vi "Read database.vi"(5 "String":string) -> (0 "error out":errorcluster, 2 "DB Data":T1)   [LabVIEW 2015]
uses:
  <vilib>/addons/database/Connection.llb/DB Tools Open Connec (String).vi
  Galobal variable_TI.vi
  <vilib>/addons/database/_DB Variant To Data/Database Variant To Data.xnode
  <vilib>/addons/database/NI_Database_API.lvlib
panel:
  out "appended array 4":string[](array[string])
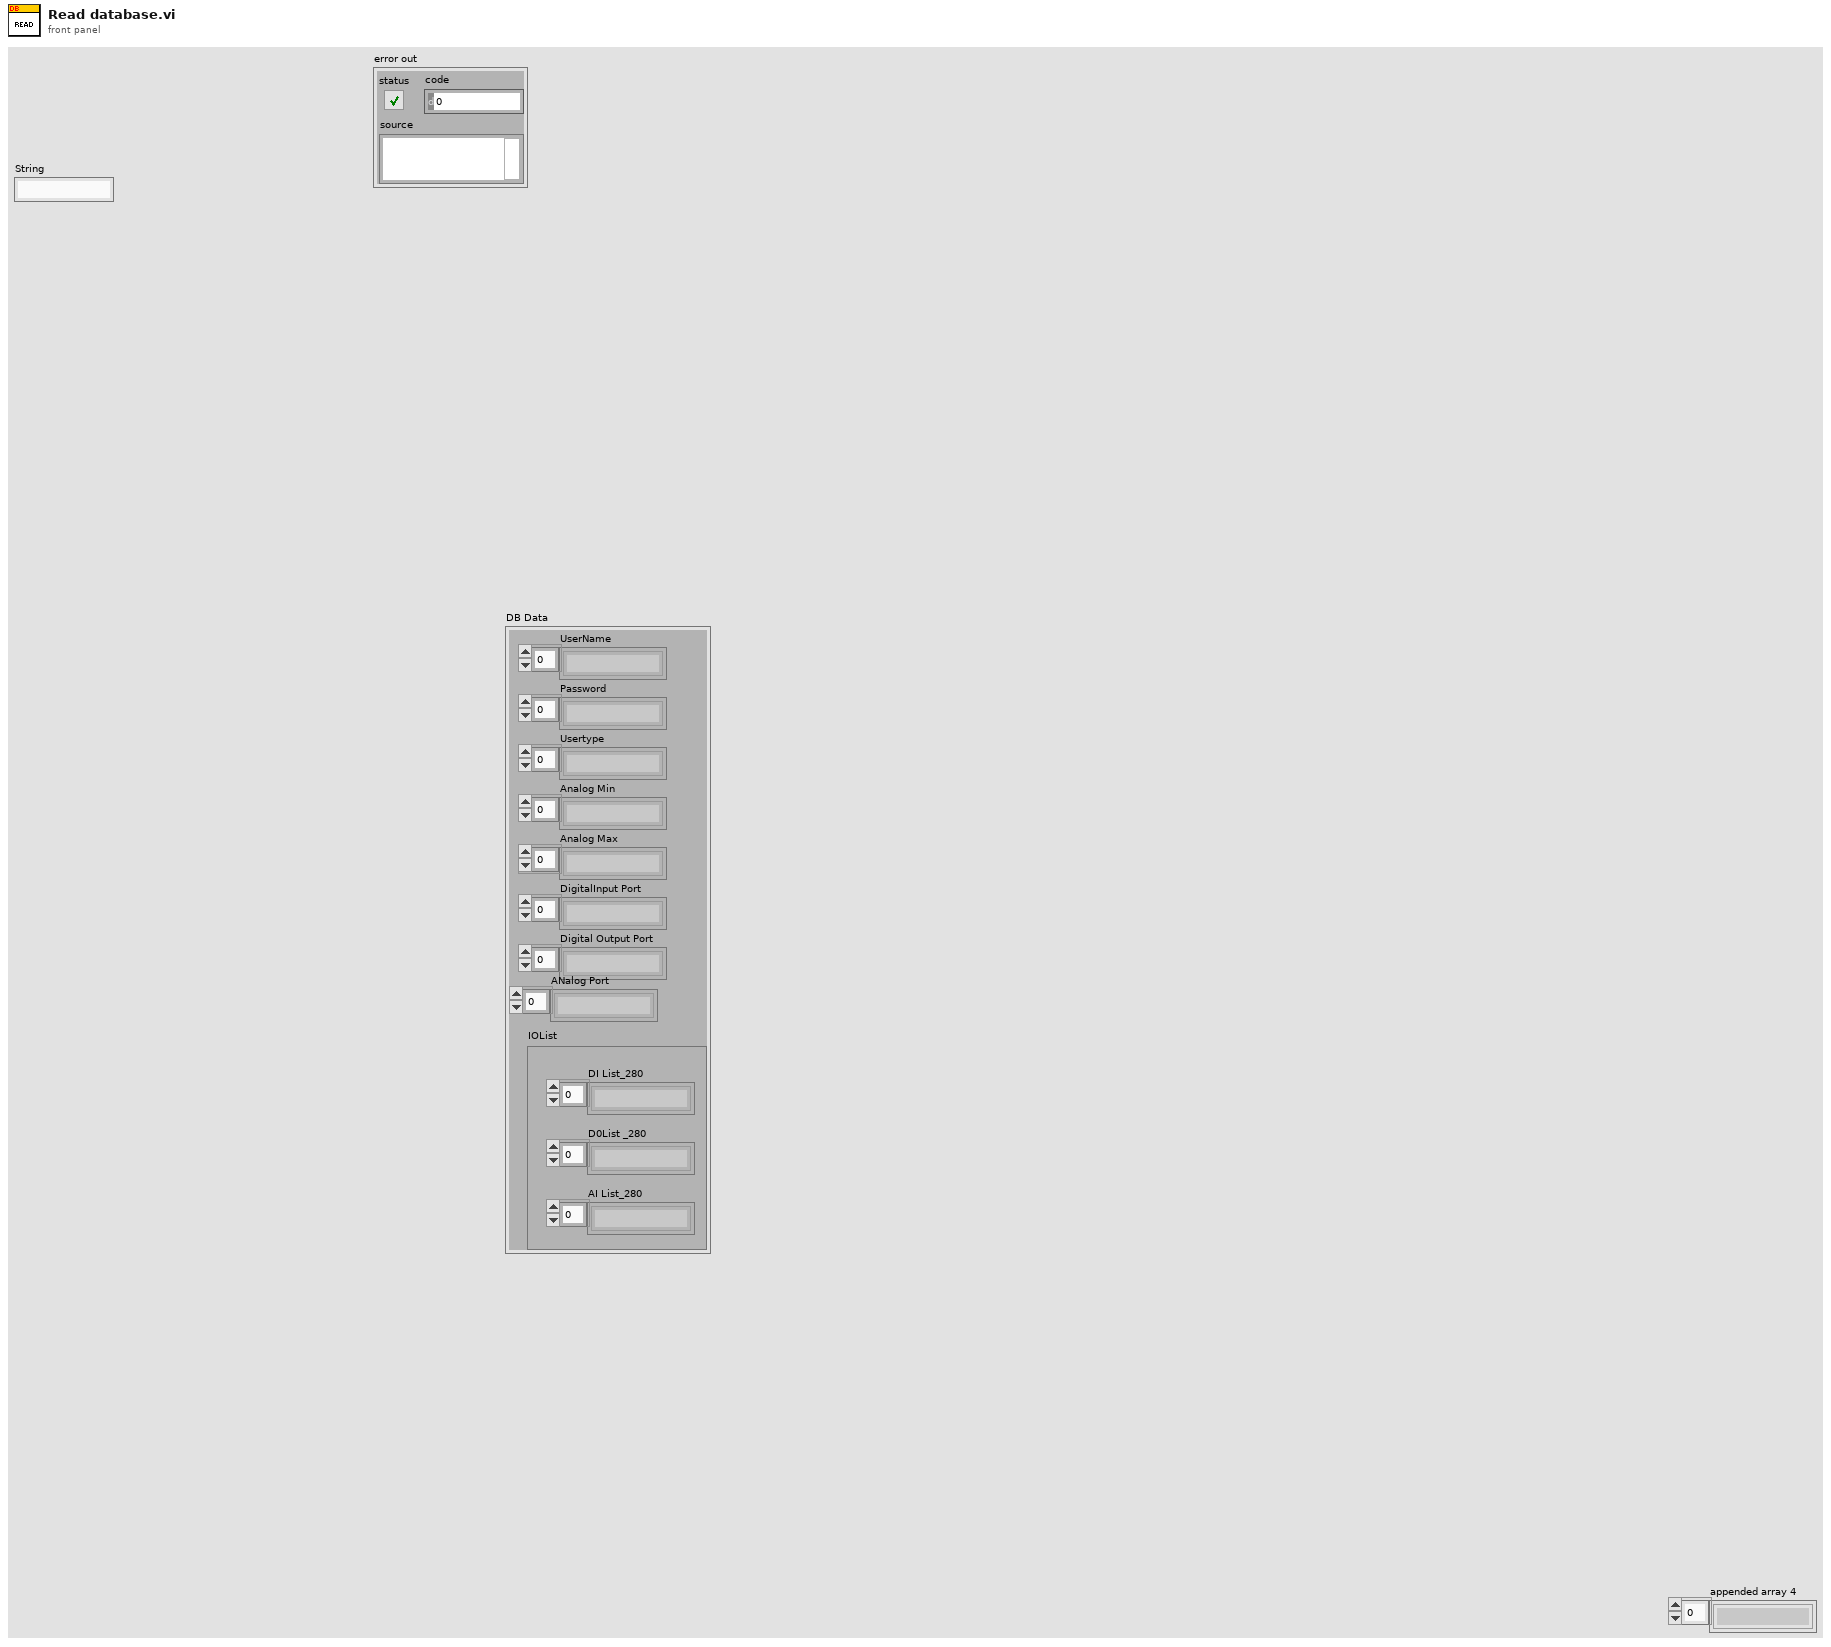
[diagram p1: front panel]
types:
  T1 = cluster{"UserName":string[], "Password":string[], "Usertype":string[], "Analog Min":string[], "Analog Max":string[], "DigitalInput Port":string[], "Digital Output Port":string[], "ANalog Port":string[], "IOList":cluster{"DI List_280":string[], "D0List _280":string[], "AI List_280":string[]}}
  T2 = cluster{"To-A":timestamp, "From-A":timestamp, "From-B":timestamp, "To-B":timestamp, "From-C":timestamp, "To-C":timestamp, "Shift":string}[]
  T3 = typedef "NI_Database_API.lvlib/Conn ObjectReference.ctl" = refnum<k1>
  T4 = cluster{"DI List_280":string[], "D0List _280":string[], "AI List_280":string[]}
  T5 = cluster{"To-A":timestamp, "From-A":timestamp, "From-B":timestamp, "To-B":timestamp, "From-C":timestamp, "To-C":timestamp, "Shift":string}
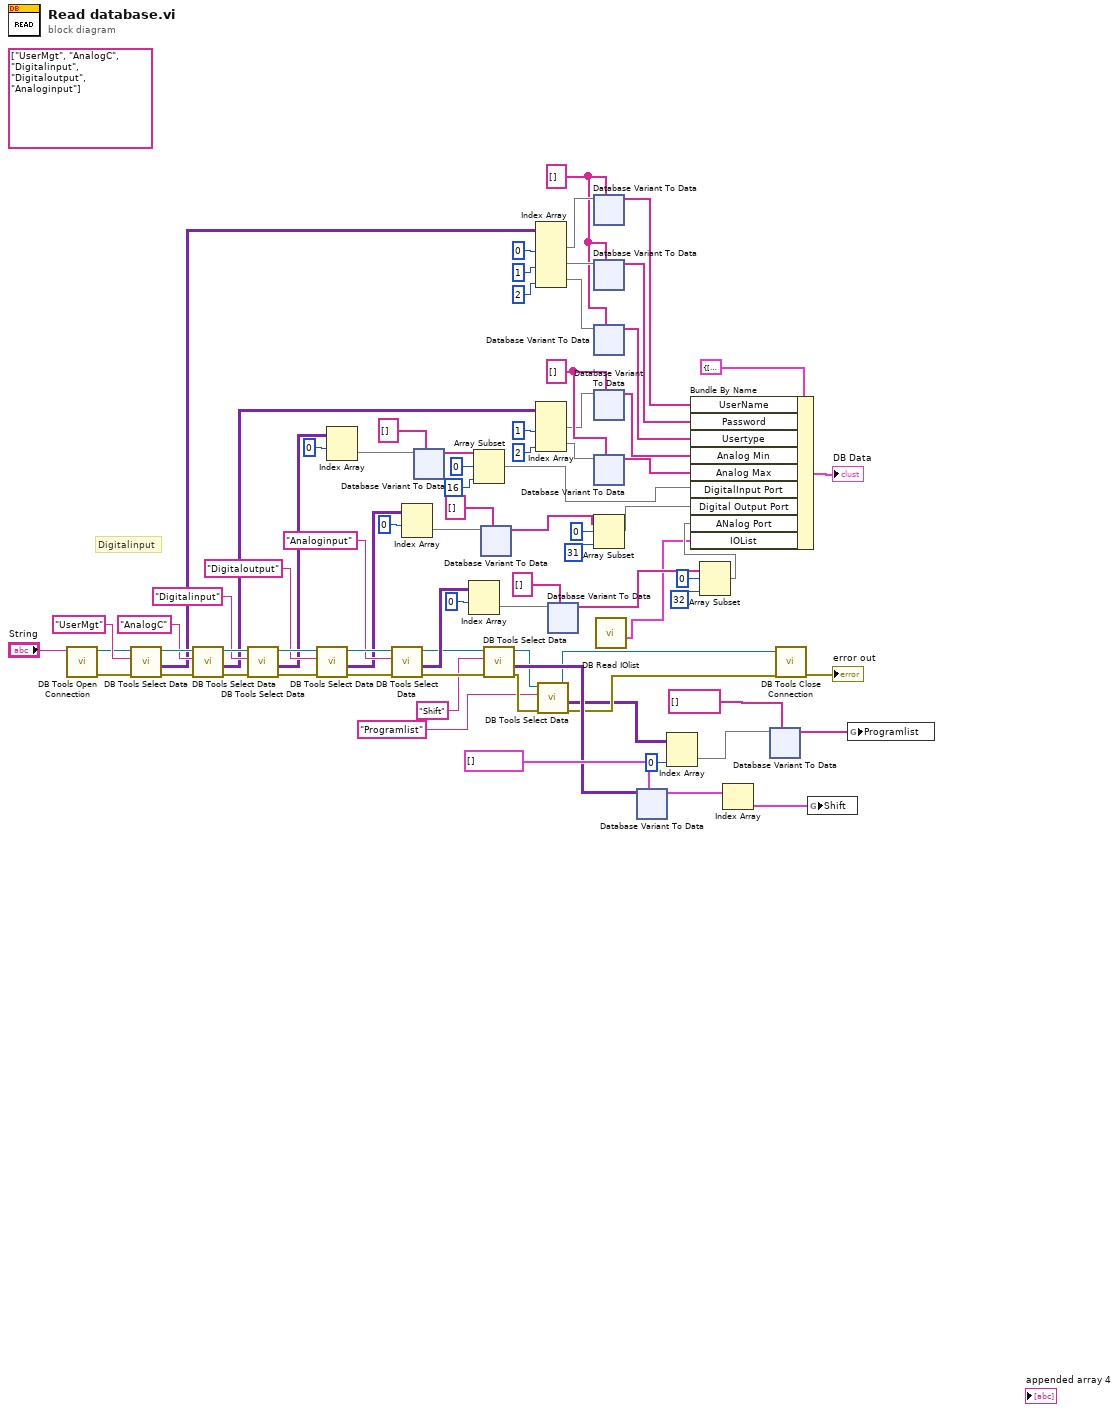
[diagram p0: block diagram]
diagram:
  w71 = string[] []
  (unwired) string[] ["UserMgt", "AnalogC", "Digitalinput", "Digitaloutput", "Analoginput"]
  w60 = string[] []
  # "Digitalinput"
  n1 = call-poly <vilib>:"DB Tools Open Connection.vi"("connection information"="String") -> ("error out"=w38:errorcluster, "connection reference"=w39:T3)  [unwired: 7 in]
  n2 = call <vilib>:"DB Tools Select Data.vi"("error in (no error)"=w38, "table"="UserMgt", "connection reference"=w39) -> ("error out"=w52:errorcluster, "data"=w37:variant[][], "connection reference out"=w50:T3)  [unwired: 3 in]
  n3 = call <vilib>:"DB Tools Select Data.vi"("error in (no error)"=w52, "table"="AnalogC", "connection reference"=w50) -> ("error out"=w51:errorcluster, "data"=w36:variant[][], "connection reference out"=w49:T3)  [unwired: 3 in]
  n4 = call <vilib>:"DB Tools Select Data.vi"("error in (no error)"=w51, "table"="Digitalinput", "connection reference"=w49) -> ("error out"=w45:errorcluster, "data"=w35:variant[][], "connection reference out"=w44:T3)  [unwired: 3 in]
  n5 = call <vilib>:"DB Tools Select Data.vi"("error in (no error)"=w45, "table"="Digitaloutput", "connection reference"=w44) -> ("error out"=w41:errorcluster, "data"=w34:variant[][], "connection reference out"=w42:T3)  [unwired: 3 in]
  n6 = Index Array(array=w35, index (row)=0 ("disabled index (col)")) -> (element=w73:variant[])  [unwired: 1 in]
  n7 = call <vilib>:"DB Tools Select Data.vi"("error in (no error)"=w41, "table"="Analoginput", "connection reference"=w42) -> ("error out"=w28:errorcluster, "data"=w33:variant[][], "connection reference out"=w27:T3)  [unwired: 3 in]
  n8 = Index Array(array=w34, index (row)=0 ("disabled index (col)")) -> (element=w74:variant[])  [unwired: 1 in]
  n9 = xnode "Database Variant To Data"("database variant"=w73, "type"=string[] []) -> ("data"=w23:string[])  [unwired: 1 in, 1 out]
  n10 = Index Array(array=w33, index (row)=0 ("disabled index (col)")) -> (element=w77:variant[])  [unwired: 1 in]
  n11 = Array Subset(array=w23, index=0, length=16) -> (w20:string[])
  n12 = xnode "Database Variant To Data"("database variant"=w74, "type"=string[] []) -> ("data"=w18:string[])  [unwired: 1 in, 1 out]
  n13 = call <vilib>:"DB Tools Select Data.vi"("error in (no error)"=w28, "table"="Shift", "connection reference"=w27) -> ("error out"=w9:errorcluster, "data"=w25:variant[][], "connection reference out"=w10:T3)  [unwired: 3 in]
  n14 = Index Array(array=w37, index (col) #1=0 ("disabled index (col)"), index (col) #2=1 ("index (col)"), index (col) #3=2 ("index (col)")) -> (element #1=w64:variant[], element #2=w61:variant[], element #3=w59:variant[])  [unwired: 3 in]
  n15 = Index Array(array=w36, index (col) #1=1 ("disabled index (col)"), index (col) #2=2 ("index (col)")) -> (element #1=w69:variant[], element #2=w70:variant[])  [unwired: 2 in]
  n16 = call <vilib>:"DB Tools Select Data.vi"("error in (no error)"=w9, "table"="Programlist", "connection reference"=w10) -> ("error out"=w6:errorcluster, "data"=w5:variant[][], "connection reference out"=w7:T3)  [unwired: 3 in]
  n17 = xnode "Database Variant To Data"("database variant"=w77, "type"=string[] []) -> ("data"=w13:string[])  [unwired: 1 in, 1 out]
  n18 = xnode "Database Variant To Data"("database variant"=w64, "type"=w60) -> ("data"=w58:string[])  [unwired: 1 in, 1 out]
  n19 = xnode "Database Variant To Data"("database variant"=w61, "type"=w60) -> ("data"=w57:string[])  [unwired: 1 in, 1 out]
  n20 = xnode "Database Variant To Data"("database variant"=w59, "type"=w60) -> ("data"=w56:string[])  [unwired: 1 in, 1 out]
  n21 = xnode "Database Variant To Data"("database variant"=w69, "type"=w71) -> ("data"=w55:string[])  [unwired: 1 in, 1 out]
  n22 = xnode "Database Variant To Data"("database variant"=w70, "type"=w71) -> ("data"=w54:string[])  [unwired: 1 in, 1 out]
  n23 = Array Subset(array=w18, index=0, length=31) -> (w16:string[])
  n24 = call "DB Read IOlist.vi"() -> ("output cluster"=w11:T4)  [unwired: 11 in]
  n25 = xnode "Database Variant To Data"("database variant"=w25, "type"=T2 []) -> ("data"=w29:T2)  [unwired: 1 in, 1 out]
  n26 = Index Array(array=w5, index (col)=0 ("disabled index (col)")) -> (element=w4:variant[])  [unwired: 1 in]
  n27 = Array Subset(array=w13, index=0, length=32) -> (w12:string[])
  n28 = Bundle By Name(cluster=T1 {"UserName"=[], "Password"=[], "Usertype"=[], "Analog Min"=[], "Analog Max"=[], "DigitalInput Port"=[], "Digital Output Port"=[], "ANalog Port"=[], "IOList"={"DI List_280"=[" Start PB (P0.0) ", "Emergency Stop (P0.1)", "Reset PB (P0.2)", "Home PB (P0.3)", "Main Pressure Signal (P0.4)", "Safety Signal-1 (P0.5)", "Safety Signal-2 (P0.6)", "Fixture Sliding Servo Home RS (P0.7)", "Fixture Sliding Servo Fault Signal (P0.8)", "LCD pressing Servo Home RS (P0.9)", "LCD pressing Servo fault Signal (P0.10)", "Spare", "Spare", "Spare", "Spare", "Model conformation PX-1 (AI2)", "Model conformation PX-2 (AI3)", "Diffuser height checking Sensor-1 (AI4)", "Diffuser height checking Sensor-2 (AI5)", "Panel Door Open Signal (AI6)", "Component CNF Sensor on Ionizer (AI7)", "Bi-adhesive tube Waste Collection bin CNF Sensor (AI8)", "Photo Prism presence Sensor (AI9)", "Lightbox presence CNF Sensor (AI10)", "Diffuser presence CNF Sensor (AI11)", "Photo prism height checking UP CYL Rs (AI12)", "Photo prism height checking DWN CYL  Rs (AI13)", "Camera slide Cyl Fwd Rs (AI14)", "Camera slide Cyl Rev Rs (AI15)", "LCD Display Rotating Unit Actuator Cyl CW PX (AI16)", "LCD Display Rotating Unit Actuator Cyl CCW PX (AI17)", "Fixture clamping Cyl Fwd Rs (AI18)", "Fixture clamping Cyl Rev Rs (AI19)", "Clip pulling unit Cyl Fwd Rs (AI20)", "Clip pulling unit Cyl Rev Rs (AI21)", "Clip clamp unit Cyl Fwd Rs (A22)", "Clip clamp unit Cyl Rev Rs (AI23)", "Barcode Scanner Ready Signal (AI24)", "Spare", "Spare", "Spare", "Spare", "Spare", "Spare", "Spare"], "D0List _280"=["Ionizer ON Sol (P0.16)", "Fixture Slide Servo Fault Reset (P0.17)", "LCD pressing servo Fault Reset (P0.18)", "Fixture Slide servo Brake ON Cmd (P0.19)", "Fixture Slide Servo Direction Command (P0.20)", "LCD pressing Servo Direction Command (P0.21)", "LCD pressing Servo Brake ON Cmd (P0.22)", "Photo prism height checking UP CYL Sol (P0.23)", "Photo prism height checking DWN CYL  Sol (P0.24)", "Camera slide Cyl Fwd Sol (P0.25)", "Camera slide Cyl Rev Sol (P0.26)", "LCD Display Rotating Unit Actuator Cyl CW Sol (P0.27)", "LCD Display Rotating Unit Actuator Cyl CCW Sol (P0.28)", "Fixture clamping Cyl Fwd Sol (P0.29)", "Fixture clamping Cyl Rev Sol (P0.30)", "Clip pulling unit Cyl Fwd Sol (P0.31)", "Clip pulling unit Cyl Rev Sol (P1.0)", "Clip clamp unit Cyl Up Sol (P1.1)", "Clip clamp unit Cyl Dwn Sol (P1.2)", "Optional required based Barcode Trigger Cmd (P1.3)", "TWL Red /Fault with Buzzer (P1.4)", "TWL Green/OK (P1.5)", "TWL Yellow/ Running (P1.6)", "Spare", "Spare", "Spare", "Spare", "Spare", "Fixture Slide Servo Pulse Command (P2.4)", "LCD pressing Servo Pulse Command (P2.5)", "Spare", "Spare"], "AI List_280"=["Loadcell Signal For LCD PRESSING (AI0)", "LVDT SIGNAL FOR PHOTO PRISM HEIGHT CHECK (AI1)"]}} ("DB Data 2"), "UserName"=w58, "Password"=w57, "Usertype"=w56, "Analog Min"=w55, "Analog Max"=w54, "DigitalInput Port"=w20, "Digital Output Port"=w16, "ANalog Port"=w12, "IOList"=w11) -> (→"DB Data":T1)
  n29 = Index Array(array=w29) -> (element=w24:T5)  [unwired: 1 in]
  n30 = xnode "Database Variant To Data"("database variant"=w4, "type"=string[] []) -> ("data"=w2:string[])  [unwired: 1 in, 1 out]
  n31 = call <vilib>:"DB Tools Close Connection.vi"("error in (no error)"=w6, "connection reference"=w7) -> ("error out"=→"error out":errorcluster)  [unwired: 5 in]
  n32 = global write "Galobal variable_TI.vi" "Shift"(w24) -> ()
  n33 = global write "Galobal variable_TI.vi" "Programlist"(w2) -> ()
